vi "LdtE200Log.vi"() -> ()   [LabVIEW 2011]
uses:
  <vilib>/Platform/TimedLoop/XDataNode/timing_clust.ctl
  <vilib>/Platform/TimedLoop/XDataNode/nitl_modes.ctl
  <vilib>/Platform/TimedLoop/XDataNode/wakeup.ctl
  <vilib>/addons/database/Connection.llb/DB Tools Open Connec (String).vi
  <vilib>/Platform/TimedLoop/XDataNode/XDataNode.xnode
  <vilib>/addons/database/NI_Database_API.lvlib
  <vilib>/Platform/TimedLoop/XDataNode/XDNodeRunTimeDep.lvlib
panel:
  in  "[s]":i64=10
  in  "stop":bool
  out "timestamp":timestamp
  out "Error Status Word":string
  out "Self-Test":string
  in  "Baud Rate":u16(ring)=2 items=["2400", "4800", "9600", "19200"]
  out "Serial Port":string
  out "Pump Power Level":u8
  out "Cutoff/°C":dbl format="%.2f"
  out "Bath temperature/°C":dbl format="%.2f"
  out "Setpoint/°C":dbl format="%.2f"
  out "Error Message":string="No Error"
  out "Instrument Identity":string
  out "error out":errorcluster
  in  "Serial Port":u16(ring) items=["Com 1", "Com 2", "Com 3", "Com 4"]
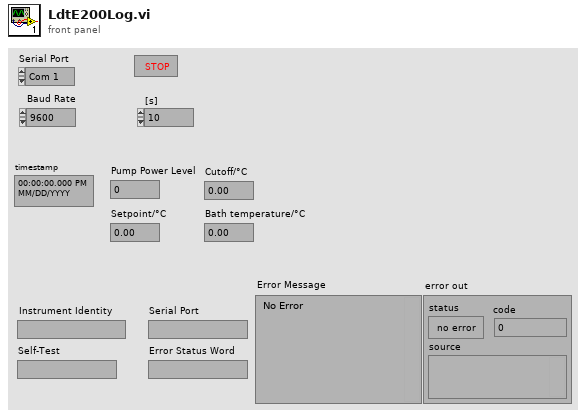
[diagram p1: front panel]
types:
  T1 = typedef "NI_Database_API.lvlib/Conn ObjectReference.ctl" = refnum<k1>
  T2 = typedef "XDNodeRunTimeDep.lvlib/timing_clust.ctl" = cluster{"Expected End [f-1]":u64, "Actual End [f-1]":u64, "Finished Late? [f-1]":bool, "Expected End [i-1]":u64, "Actual End [i-1]":u64, "Finished Late? [i-1]":bool, "Expected Start [i]":u64, "Actual Start [i]":u64, "Expected Start [f]":u64, "Actual Start [f]":u64, "Source Name":string, "Structure Name":string, "Period":i64, "Deadline":i64, "Offset":i64, "Start":i64, "Priority":i32, "Timeout":i32, "Mode":T3, "Wakeup Reason":T4, "Error":errorcluster, "Source Type":string, "Secondary Source Type":string, "Global End Time":u64, "Global Start Time":u64, "Frame Duration":u64, "Iteration Duration":u64, "Assigned CPU":i32, "I/O Scan Engine Mode":u32}
  T3 = typedef "XDNodeRunTimeDep.lvlib/nitl_modes.ctl" = enum32{"No Change", "Process missed periods, maintain original phase", "Discard missed periods, maintain original phase", "Process missed periods, ignore original phase", "Discard missed periods, ignore original phase"}
  T4 = typedef "XDNodeRunTimeDep.lvlib/wakeup.ctl" = enum32{"Normal", "Aborted", "Asynchronous wakeup", "Timing source error", "Timed loop error", "Timeout"}
  T5 = cluster{"seconds since 1Jan1904":timestamp, "Pump Power Level":u8, "Setpoint Temperature":dbl, "Cutoff Temperature":dbl, "Internal Bath Temperature":dbl}
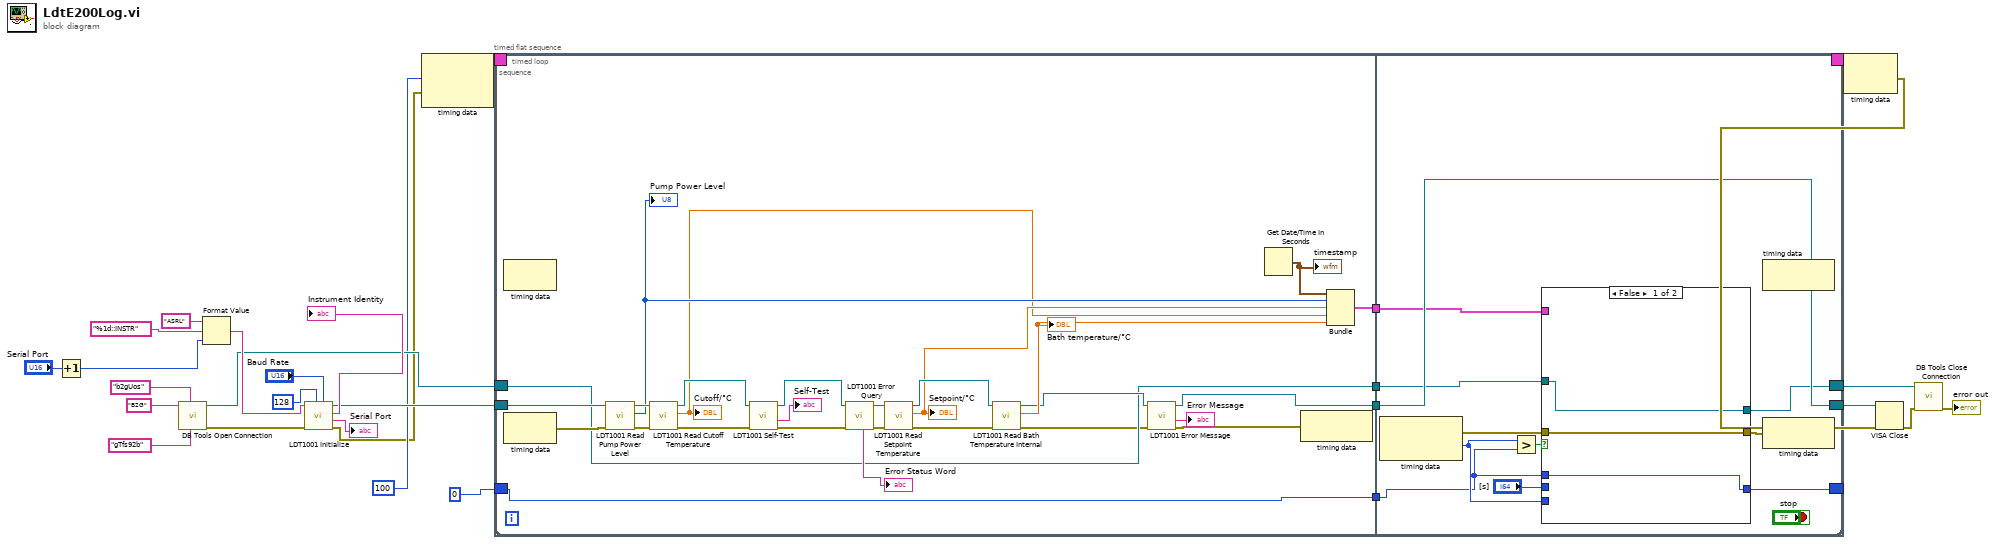
[diagram p0: block diagram]
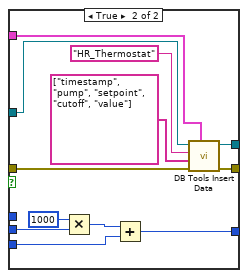
[diagram p2: hidden frame]
diagram:
  n1 = Increment(x="Serial Port") -> (x+1=w17:u16)
  n2 = call-poly <vilib>:"DB Tools Open Connection.vi"("password"="gTfs92b", "userID"="b2gUos", "connection information"="B2G") -> ("error out"=w12:errorcluster, "connection reference"=w15:T1)  [unwired: 5 in]
  n3 = Format Value(string ("")="ASRL", format string="%1d::INSTR", value (0)=w17) -> (output string=w20:string)
  n4 = call <instrlib>:"LDT1001 Initialize.vi"("Baud Rate (2: 9600 default)"="Baud Rate", "RS485 Instrument Address (128: RS232 default)"=u32 128 ("RS485 Addr. (128: RS232)"), "error in (no error)"=w12, "Instrument Descriptor (ASRL1::INSTR)"=w20) -> ("error out"=w3:errorcluster, "Serial Port"=→"Serial Port":string, "Instrument Identity"=→"Instrument Identity":string, "VISA session"=w11:refnum<visa-resource-name>)  [unwired: 4 in]
  n5 = node-c288(i64 100 ("Period"), w3) -> (w6:T2)
  n6 = timed-loop {
    shift-right: [w30] -> w23
    shift-left: w11 -> [w31]
    shift-right: [w28] -> w7
    shift-left: w15 -> [w29]
    timing: w6 -> [_]
    timing-out: [_] -> w5
    shift-right: [w27] -> _
    shift-left: i64 0 ("Actual Start [f]") -> [w26]
    stop <- "stop" stop-if-true
    n7 = timed-sequence {
      timing: _ -> [_]
      timing-out: _ -> [_]
      tunnel: w31 -> [w41]
      tunnel: [w40] -> w30
      tunnel: w29 -> [w39]
      tunnel: [w38] -> w28
      tunnel: [w34] -> w27
      tunnel: w26 -> [w32]
      n8 = timed-flat-sequence {
        tunnel: w41 -> [w68]
        tunnel: w39 -> [w45]
        tunnel: [w67] -> w37
        tunnel: [w45] -> w36
        tunnel: [w43] -> w35
        tunnel: [w42] -> w33
        tunnel: w32 -> [w42]
        tunnel: [w84] -> w38
        tunnel: [w85] -> w40
        tunnel: w37 -> [w85]
        tunnel: w36 -> [w83]
        tunnel: w35 -> [w82]
        tunnel: [w78] -> w34
        tunnel: w33 -> [w74]
        frame #0 {
          n9 = node-c288() -> (w48:errorcluster)  [unwired: 1 in]
          n10 = call <instrlib>:"LDT1001 Read Pump Power Level.vi"("error in (no error)"=w48, "VISA session"=w68) -> ("error out"=w56:errorcluster, "Pump Power Level"=w55:u8, "dup VISA session"=w57:refnum<visa-resource-name>)  [unwired: 7 in]
          "Pump Power Level" <- w55
          n11 = call <instrlib>:"LDT1001 Read Cutoff Temperature.vi"("error in (no error)"=w56, "VISA session"=w57) -> ("error out"=w58:errorcluster, "Cutoff Temperature"=w53:dbl, "dup VISA session"=w59:refnum<visa-resource-name>)  [unwired: 7 in]
          "Cutoff/°C" <- w53
          n12 = call <instrlib>:"LDT1001 Self-Test.vi"("error in (no error)"=w58, "VISA session"=w59) -> ("error out"=w50:errorcluster, "Self-Test Response"=→"Self-Test":string, "dup VISA session"=w49:refnum<visa-resource-name>)  [unwired: 6 in, 1 out]
          n13 = call <instrlib>:"LDT1001 Error Query.vi"("error in (no error)"=w50, "VISA session"=w49) -> ("error out"=w62:errorcluster, "dup VISA session"=w63:refnum<visa-resource-name>, "Error Status Word"=→"Error Status Word":string)  [unwired: 5 in, 2 out]
          n14 = call <instrlib>:"LDT1001 Read Setpoint Temperature.vi"("error in (no error)"=w62, "VISA session"=w63) -> ("error out"=w66:errorcluster, "Setpoint Temperature"=w54:dbl, "dup VISA session"=w65:refnum<visa-resource-name>)  [unwired: 7 in]
          "Setpoint/°C" <- w54
          n15 = call <instrlib>:"LDT1001 Read Bath Temperature Internal.vi"("error in (no error)"=w66, "VISA session"=w65) -> ("error out"=w44:errorcluster, "Internal Bath Temperature"=w52:dbl, "dup VISA session"=w46:refnum<visa-resource-name>)  [unwired: 7 in]
          "Bath temperature/°C" <- w52
          n16 = call <instrlib>:"LDT1001 Error Message.vi"("error in (no error)"=w44, "VISA session"=w46) -> ("error out"=w47:errorcluster, "Error Message (empty)"=→"Error Message":string, "dup VISA session"=w67:refnum<visa-resource-name>)  [unwired: 5 in, 2 out]
          n17 = Get Date/Time In Seconds() -> (seconds since 1Jan1904=w51:timestamp)
          "timestamp" <- w51
          n18 = node-c288(w47) -> ()  [unwired: 1 out]
          n19 = Bundle("seconds since 1Jan1904"=w51, "Pump Power Level"=w55, "Setpoint Temperature"=w54, "Cutoff Temperature"=w53, "Internal Bath Temperature"=w52) -> (w43:T5)  [unwired: 1 in]
        }
        frame #1 {
          n20 = node-c288() -> (w81:errorcluster, w77:i64)  [unwired: 1 in]
          n21 = Greater?(x=w77, y=w74) -> (0:w76:bool)
          n22 = case shown="False" w76 {
            tunnel: [w86 w100] -> w84
            tunnel: w83 -> [w86 w99]
            tunnel: w82 -> [_ w97]
            tunnel: w81 -> [w88 w95]
            tunnel: [w88 w94] -> w80
            tunnel: [w87 w91] -> w78
            tunnel: w77 -> [_ w89]
            tunnel: "[s]" -> [_ w90]
            tunnel: w74 -> [w87 _]
            frame False {
            }
            frame True {
              n23 = Multiply(x=i64 1000, y=w90) -> (x*y=w93:i64)
              n24 = Add(x=w93, y=w89) -> (x+y=w91:i64)
              n25 = call <vilib>:"DB Tools Insert Data.vi"("data"=w97, "error in (no error)"=w95, "columns"=string[] ["timestamp", "pump", "setpoint", "cutoff", "value"], "table"="HR_Thermostat", "connection reference"=w99) -> ("error out"=w94:errorcluster, "connection reference out"=w100:T1)  [unwired: 5 in]
            }
          }
          n26 = node-c288(w80) -> ()  [unwired: 1 out]
        }
      }
    }
    n27 = node-c288() -> ()  [unwired: 1 in, 1 out]
    n28 = node-c288() -> ()  [unwired: 1 in, 1 out]
  }
  n29 = node-c288(w5) -> (w2:errorcluster)
  n30 = VISA Close(VISA resource name=w23, error in (no error)=w2) -> (error out=w9:errorcluster)
  n31 = call <vilib>:"DB Tools Close Connection.vi"("error in (no error)"=w9, "connection reference"=w7) -> ("error out"=→"error out":errorcluster)  [unwired: 5 in]
